vi "myRIO_BRig SPI Output Logic.vi"(6 "Enable?":bool, 9 "Sample on trailing edge (Phase)?":bool, 10 "Falling edge leads (Polarity)?":bool, 11 "State":T1) -> (0 "Increment?":bool, 1 "Setup?":bool, 2 "Sample?":bool, 3 "SCLK":bool)   [LabVIEW 2014]
uses:
  myRIO_BRig SPI States.ctl
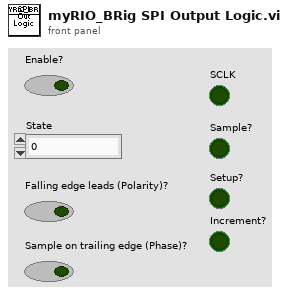
[diagram p1: front panel]
types:
  T1 = typedef "myRIO_BRig SPI States.ctl" = fxp<+,3,3>
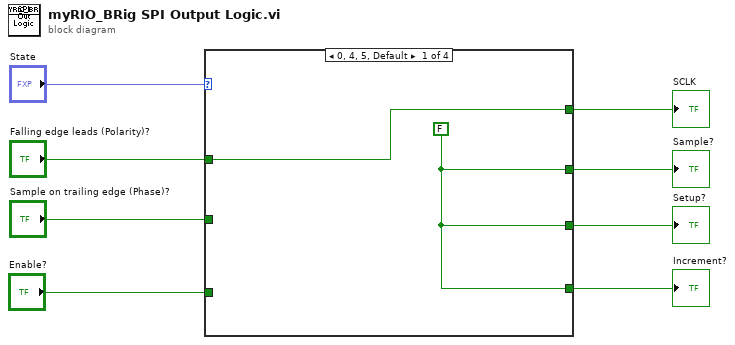
[diagram p0: block diagram]
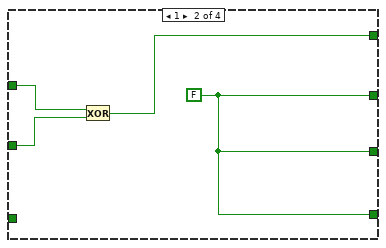
[diagram p2: hidden frame]
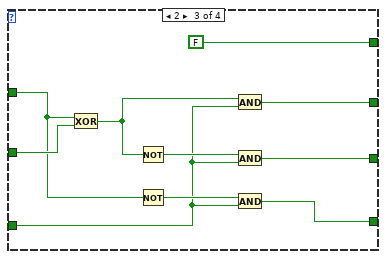
[diagram p3: hidden frame]
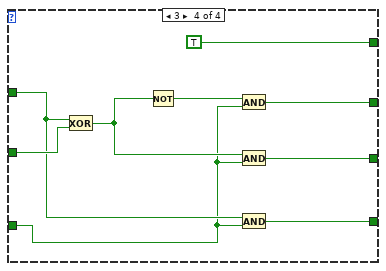
[diagram p4: hidden frame]
diagram:
  n1 = case shown="0, 4, 5, Default" "State" {
    tunnel: "Falling edge leads (Polarity)?" -> [w10 w14 w16 w27]
    tunnel: "Sample on trailing edge (Phase)?" -> [_ w13 w23 w32]
    tunnel: [w10 w12 FALSE ("Polarity?") TRUE ("Polarity?")] -> w6
    tunnel: "Enable?" -> [_ _ w15 w25]
    tunnel: [w9 w11 w22 w30] -> w5
    tunnel: [w9 w11 w20 w28] -> w4
    tunnel: [w9 w11 w17 w26] -> w3
    frame 0, 4, 5, Default {
      w9 = FALSE ("Polarity?")
    }
    frame 1 {
      w11 = FALSE ("Polarity?")
      n2 = Exclusive Or(1:w13, 2:w14) -> (0:w12:bool)
    }
    frame 2 {
      n3 = Exclusive Or(1:w23, 2:w16) -> (0:w19:bool)
      n4 = Not(x=w19) -> (.not. x?=w21:bool)
      n5 = Not(x=w16) -> (.not. x?=w18:bool)
      n6 = And(x=w19, y=w15) -> (x .and. y?=w22:bool)
      n7 = And(x=w21, y=w15) -> (x .and. y?=w20:bool)
      n8 = And(x=w18, y=w15) -> (x .and. y?=w17:bool)
    }
    frame 3 {
      n9 = Exclusive Or(1:w32, 2:w27) -> (0:w29:bool)
      n10 = Not(x=w29) -> (.not. x?=w31:bool)
      n11 = And(x=w31, y=w25) -> (x .and. y?=w30:bool)
      n12 = And(x=w29, y=w25) -> (x .and. y?=w28:bool)
      n13 = And(x=w27, y=w25) -> (x .and. y?=w26:bool)
    }
  }
  "SCLK" <- w6
  "Sample?" <- w5
  "Increment?" <- w3
  "Setup?" <- w4
